vi "Terminal_Global_pressure_display.vi"   [LabVIEW 2014]
types:
  T1 = cluster{"径向油缸加载压力":u16, "轴向油缸加载压力":u16, "油箱1油液温度":u16, "润滑油温度":u16, "油箱2油液温度":u16, "试验轴承供油压力":u16, "试验轴承供油流量":u16, "陪试轴承供油流量":u16, "陪试轴承供油压力":u16, "陪试轴承供油温度":u16, "液压子系统状态字":cluster{"加载单元":cluster{"供油过滤器堵塞报警":bool, "回油过滤器堵塞报警":bool, "液位过高报警":bool, "液位过低报警":bool}, "试验轴承单元":cluster{"加热装置异常报警":bool, "油箱1液位过高报警":bool, "油箱1液位过低报警":bool, "油箱2液位过高报警":bool, "油箱2液位过低报警":bool, "供油过滤器堵塞报警":bool, "循环回路过滤器堵塞报警":bool, "回油过滤器堵塞报警":bool}, "陪试轴承单元":cluster{"供油过滤器1堵塞报警":bool, "供油过滤器2堵塞报警":bool, "回油过滤器堵塞报警":bool, "油箱液位过高报警":bool, "油箱液位过低报警":bool}}}
  T2 = cluster{"径向油缸加载压力":u16, "轴向油缸加载压力":u16, "油箱1油液温度":u16, "润滑油温度":u16, "油箱2油液温度":u16, "试验轴承供油压力":u16, "试验轴承供油流量":u16, "陪试轴承供油流量":u16, "陪试轴承供油压力":u16, "陪试轴承供油温度":u16}
  T3 = cluster{"供油过滤器1堵塞报警":bool, "供油过滤器2堵塞报警":bool, "回油过滤器堵塞报警":bool, "油箱液位过高报警":bool, "油箱液位过低报警":bool}
  T4 = cluster{"供油过滤器堵塞报警":bool, "回油过滤器堵塞报警":bool, "液位过高报警":bool, "液位过低报警":bool}
  T5 = cluster{"加热装置异常报警":bool, "油箱1液位过高报警":bool, "油箱1液位过低报警":bool, "油箱2液位过高报警":bool, "油箱2液位过低报警":bool, "供油过滤器堵塞报警":bool, "循环回路过滤器堵塞报警":bool, "回油过滤器堵塞报警":bool}
  T6 = cluster{"油箱1油液温度":dbl, "油箱2油液温度":dbl, "供油压力最小值":dbl, "供油压力最大值":dbl, "润滑油温度T2最小值":dbl, "润滑油温度T2最大值":dbl, "供油流量L1最小值":dbl, "供油流量L1最大值":dbl}
  T7 = cluster{"供油压力最小值":dbl, "供油压力最大值":dbl, "试验轴承供油压力":u16}
  T8 = cluster{cluster{"油箱1油液温度":dbl, "油箱1油液温度":u16}, cluster{sgl, sgl, "润滑油温度":u16}, cluster{"油箱2油液温度":dbl, "油箱2油液温度":u16}, cluster{"供油压力最小值":dbl, "供油压力最大值":dbl, "试验轴承供油压力":u16}, cluster{sgl, sgl, "试验轴承供油流量":u16}, "试验轴承单元":cluster{"加热装置异常报警":bool, "油箱1液位过高报警":bool, "油箱1液位过低报警":bool, "油箱2液位过高报警":bool, "油箱2液位过低报警":bool, "供油过滤器堵塞报警":bool, "循环回路过滤器堵塞报警":bool, "回油过滤器堵塞报警":bool}}
  T9 = cluster{"陪试轴承供油流量":u16, "陪试轴承供油压力":u16, "陪试轴承供油温度":u16, "陪试轴承单元":cluster{"供油过滤器1堵塞报警":bool, "供油过滤器2堵塞报警":bool, "回油过滤器堵塞报警":bool, "油箱液位过高报警":bool, "油箱液位过低报警":bool}}
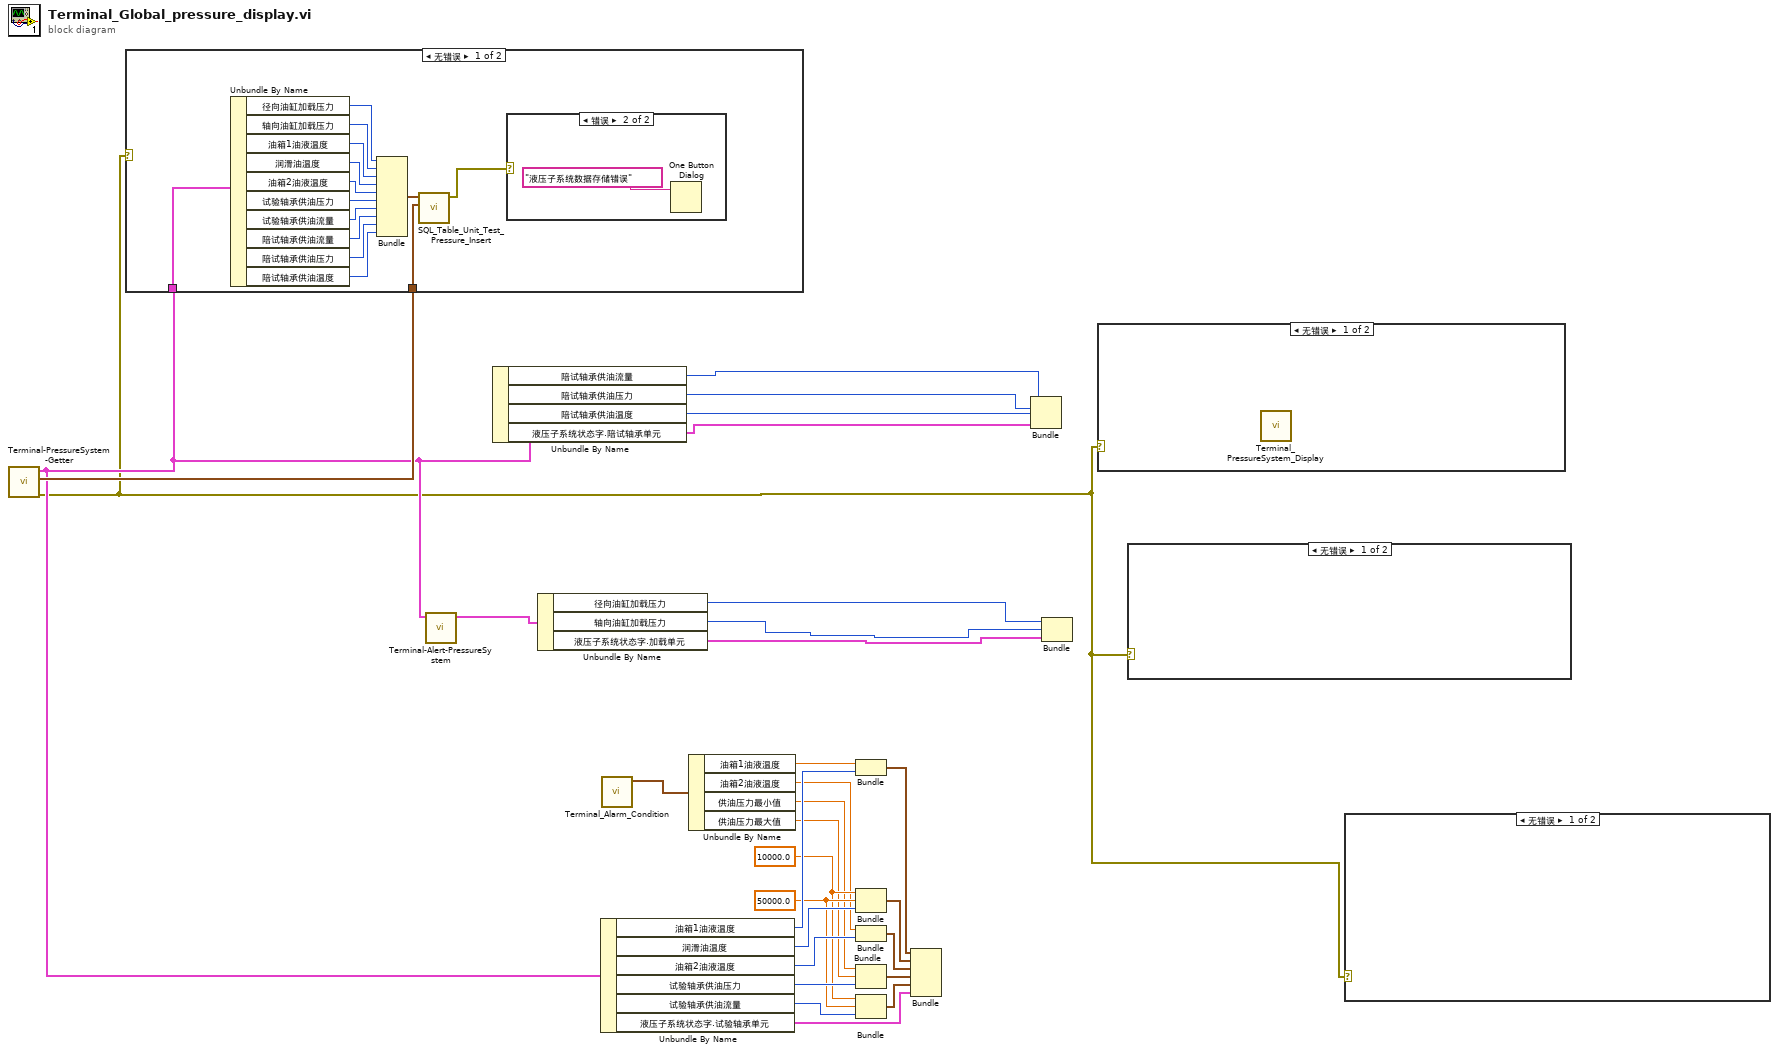
[diagram p0: block diagram]
diagram:
  w22 = sgl 50000.0
  w15 = sgl 10000.0
  n1 = call "Terminal-PressureSystem-Getter.vi"() -> ("error out"=w1:errorcluster, "时间标识"=w13:timestamp, "设备信息"=w12:T1)  [unwired: 9 in]
  n2 = case shown="无错误" w1 {
    tunnel: w13 -> [w34 _]
    tunnel: w12 -> [w32 _]
    frame No Error {
      n3 = Unbundle By Name(w32) -> ("径向油缸加载压力"=w45:u16, "轴向油缸加载压力"=w44:u16, "油箱1油液温度"=w43:u16, "润滑油温度"=w42:u16, "油箱2油液温度"=w41:u16, "试验轴承供油压力"=w40:u16, "试验轴承供油流量"=w39:u16, "陪试轴承供油流量"=w38:u16, "陪试轴承供油压力"=w37:u16, "陪试轴承供油温度"=w36:u16)
      n4 = Bundle("径向油缸加载压力"=w45, "轴向油缸加载压力"=w44, "油箱1油液温度"=w43, "润滑油温度"=w42, "油箱2油液温度"=w41, "试验轴承供油压力"=w40, "试验轴承供油流量"=w39, "陪试轴承供油流量"=w38, "陪试轴承供油压力"=w37, "陪试轴承供油温度"=w36) -> (w35:T2)  [unwired: 1 in]
      n5 = call "SQL_Table_Unit_Test_Pressure_Insert.vi"("时间标识"=w34, "液压子系统数据"=w35) -> ("error out"=w33:errorcluster)  [unwired: 9 in]
      n6 = case shown="错误" w33 {
        frame No Error {
        }
        frame Error {
          n7 = One Button Dialog(message="液压子系统数据存储错误" ("消息")) -> ()  [unwired: 1 in, 1 out]
        }
      }
    }
    frame Error {
    }
  }
  n8 = call "Terminal-Alert-PressureSystem.vi"("液压子系统设备信息"=w12) -> ("液压子系统设备信息输出"=w28:T1)  [unwired: 10 in]
  n9 = Unbundle By Name(w12) -> ("陪试轴承供油流量"=w6:u16, "陪试轴承供油压力"=w5:u16, "陪试轴承供油温度"=w4:u16, "液压子系统状态字.陪试轴承单元"=w31:T3)
  n10 = Unbundle By Name(w28) -> ("径向油缸加载压力"=w2:u16, "轴向油缸加载压力"=w3:u16, "液压子系统状态字.加载单元"=w29:T4)
  n11 = Unbundle By Name(w12) -> ("油箱1油液温度"=w27:u16, "润滑油温度"=w26:u16, "油箱2油液温度"=w25:u16, "试验轴承供油压力"=w24:u16, "试验轴承供油流量"=w23:u16, "液压子系统状态字.试验轴承单元"=w17:T5)
  n12 = call "Terminal_Alarm_Condition.vi"() -> ("试验轴承单元"=w11:T6)  [unwired: 11 in]
  n13 = Unbundle By Name(w11) -> ("油箱1油液温度"=w10:dbl, "油箱2油液温度"=w9:dbl, "供油压力最小值"=w8:dbl, "供油压力最大值"=w7:dbl)
  n14 = Bundle("油箱1油液温度"=w10, "油箱1油液温度"=w27) -> (w14:cluster{"油箱1油液温度":dbl, "油箱1油液温度":u16})  [unwired: 1 in]
  n15 = Bundle(w15, w22, "润滑油温度"=w26) -> (w21:cluster{sgl, sgl, "润滑油温度":u16})  [unwired: 1 in]
  n16 = Bundle("油箱2油液温度"=w9, "油箱2油液温度"=w25) -> (w20:cluster{"油箱2油液温度":dbl, "油箱2油液温度":u16})  [unwired: 1 in]
  n17 = Bundle("供油压力最小值"=w8, "供油压力最大值"=w7, "试验轴承供油压力"=w24) -> (w19:T7)  [unwired: 1 in]
  n18 = Bundle(w15, w22, "试验轴承供油流量"=w23) -> (w18:cluster{sgl, sgl, "试验轴承供油流量":u16})  [unwired: 1 in]
  n19 = Bundle(w14, w21, w20, w19, w18, "试验轴承单元"=w17) -> (w16:T8)  [unwired: 1 in]
  n20 = Bundle("陪试轴承供油流量"=w6, "陪试轴承供油压力"=w5, "陪试轴承供油温度"=w4, "陪试轴承单元"=w31) -> (w30:T9)  [unwired: 1 in]
  n21 = Bundle("径向油缸加载压力"=w2, "轴向油缸加载压力"=w3, "加载单元"=w29) -> ()  [unwired: 1 in, 1 out]
  n22 = case shown="无错误" w1 {
    frame No Error {
      n23 = call "Terminal_PressureSystem_Display.vi"() -> ()  [unwired: 12 in]
    }
    frame Error {
    }
  }
  n24 = case shown="无错误" w1 {
    frame No Error {
    }
    frame Error {
    }
  }
  n25 = case shown="无错误" w1 {
    frame No Error {
    }
    frame Error {
    }
  }
